vi "3-1.vi"() -> ()   [LabVIEW 2015]
panel:
  out "Cluster Array 2":cluster{"Array 2":dbl[]}[](array[cluster])
  out "Cluster Array 1":cluster{"Array 2":dbl[]}[](array[cluster])
  in  "Array 2":dbl[](array[numeric])
  in  "Array":dbl[](array[numeric])
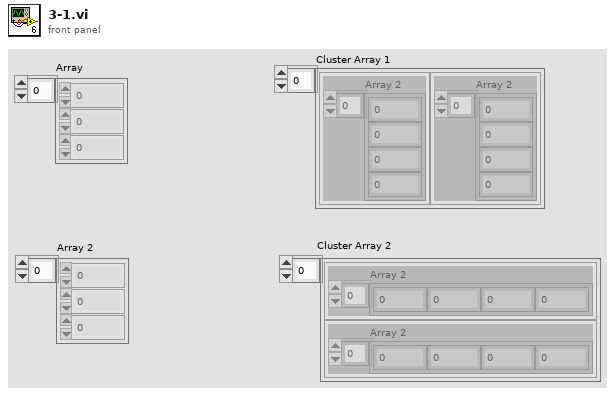
[diagram p1: front panel]
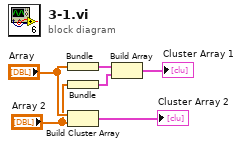
[diagram p0: block diagram]
diagram:
  n1 = Bundle("Array"="Array") -> (w6:cluster{"Array":dbl[]})  [unwired: 1 in]
  n2 = Bundle("Array 2"="Array 2") -> (w5:cluster{"Array 2":dbl[]})  [unwired: 1 in]
  n3 = Build Cluster Array("Array", "Array 2") -> (→"Cluster Array 2":cluster{"Array 2":dbl[]}[])
  n4 = Build Array(w6, w5) -> (→"Cluster Array 1":cluster{"Array 2":dbl[]}[])
